vi "On Recompile Action VI Name.vi"(11 "CD Template in":refnum<class "NIVS_PPL_Inline HW Interface.lvclass">) -> (2 "On Recompile Action VI Name":string)   [LabVIEW 2020, in "NIVS_PPL_Inline HW Interface.lvclass"]
uses:
  NIVS_PPL_Inline HW Interface.lvclass
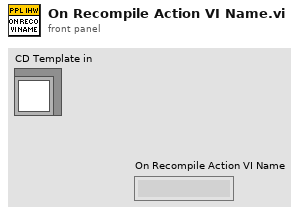
[diagram p1: front panel]
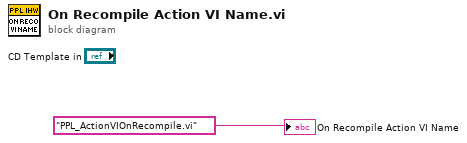
[diagram p0: block diagram]
diagram:
  "On Recompile Action VI Name" <- "PPL_ActionVIOnRecompile.vi" ("On Recompile Action VI Name")
